vi "Get Data Server Options.vi"(8 "error in":errorcluster, 11 "data sharing framework custom device in":T1 format="%.0x") -> (0 "error out":errorcluster, 1 "data server frequency (Hz)":dbl, 2 "data server enabled?":bool, 3 "data sharing framework custom device out":T1 format="%.0x", 4 "launch data viewer?":bool)   [LabVIEW 2020, in "Data Sharing Framework Custom Device Scripting.lvlib"]
doc: "Reads the <b>data server enabled?</b>, <b>data server frequency (Hz)</b>, and <b>launch data viewer?</b> options."
uses:
  Data Sharing Framework Custom Device Scripting.lvlib
  <vilib>/NI VeriStand/Custom Device API/Custom Device Item Ref.ctl
  DSF Shared.lvlib
  <vilib>/NI VeriStand/Custom Device API/Custom Device API.lvlib
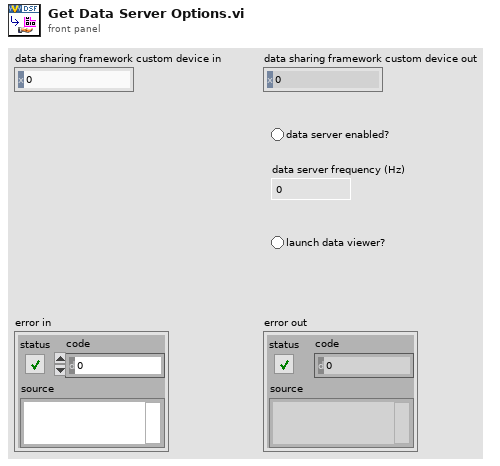
[diagram p1: front panel]
types:
  T1 = typedef "Custom Device API.lvlib/Custom Device Item Ref.ctl" = u64
  T2 = typedef "DSF Core.lvlibp/Framework.lvclass/Framework Options.ctl" = cluster{"FIFO Options":T3, "Thread Options":T4, "Plugin Options":T5, "Performance Options":T6, "Data Server Options":T7}
  T3 = typedef "DSF Core.lvlibp/Framework.lvclass/DSF FIFO Options.ctl" = cluster{"Infinite Timeouts":bool}
  T4 = typedef "DSF Core.lvlibp/Thread.lvclass/Thread Options.ctl" = cluster{"Show FP On Call":bool, "Close FP After Call":bool, "Allow Debugging":bool}
  T5 = typedef "DSF Core.lvlibp/Framework.lvclass/DSF Plugin Options.ctl" = cluster{"Default Components":bool}
  T6 = typedef "DSF Core.lvlibp/DSF Performance Options.ctl" = cluster{"Measure Period":bool, "Measure Rx/Tx Duration":bool}
  T7 = typedef "DSF Core.lvlibp/Framework.lvclass/Data Server Options.ctl" = cluster{"Enable Data Server":bool, "Period":u32}
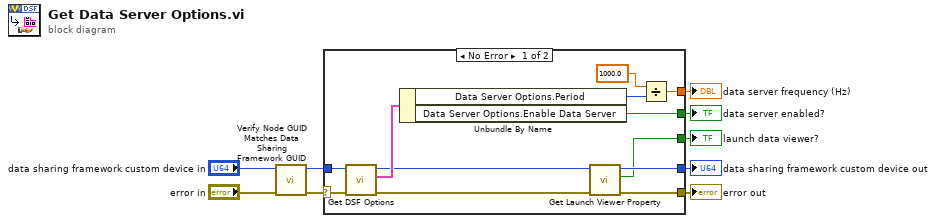
[diagram p0: block diagram]
diagram:
  n1 = call "Verify Node GUID Matches Data Sharing Framework GUID.vi"("error in"="error in", "data sharing framework custom device in"="data sharing framework custom device in") -> ("error out"=w1:errorcluster, "data sharing framework custom device out"=w2:T1)  [unwired: 8 in]
  n2 = case shown="No Error" w1 {
    selector: w1 -> [w10 w23]
    tunnel: [w17 w22] -> w9
    tunnel: [w16 w23] -> w8
    tunnel: [w14 _] -> w7
    tunnel: [w13 _] -> w6
    tunnel: [w12 _] -> w5
    tunnel: w2 -> [w11 w22]
    frame No Error {
      n3 = call "Get DSF Options.vi"("error in (no error)"=w10, "Item Ref in"=w11) -> ("error out"=w18:errorcluster, "options"=w20:T2, "Item Ref out"=w19:T1)  [unwired: 7 in]
      n4 = Unbundle By Name(w20) -> ("Data Server Options.Period"=w15:u32, "Data Server Options.Enable Data Server"=w13:bool)
      n5 = call "Get Launch Viewer Property.vi"("error in (no error)"=w18, "Item Ref in"=w19) -> ("error out"=w16:errorcluster, "launch viewer"=w12:bool, "Item Ref out"=w17:T1)  [unwired: 7 in]
      n6 = Divide(x=1000.0 ("y"), y=w15) -> (x/y=w14:dbl)
    }
    frame Error {
    }
  }
  "data sharing framework custom device out" <- w9
  "data server frequency (Hz)" <- w7
  "error out" <- w8
  "data server enabled?" <- w6
  "launch data viewer?" <- w5
